vi "Write Self-Test.vi"(8 "error in (no error)":errorcluster, 10 "Self-Test":bool, 11 "Selftest Device Msg in":refnum<class "Selftest Device Msg.lvclass">) -> (0 "error out":errorcluster, 3 "Selftest Device Msg out":refnum<class "Selftest Device Msg.lvclass">)   [LabVIEW 2016, in "CS++DeviceActor.lvlib" / "Selftest Device Msg.lvclass"]
uses:
  Selftest Device Msg.lvclass
  Selftest Device Msg.lvclass/Selftest Device Msg.ctl
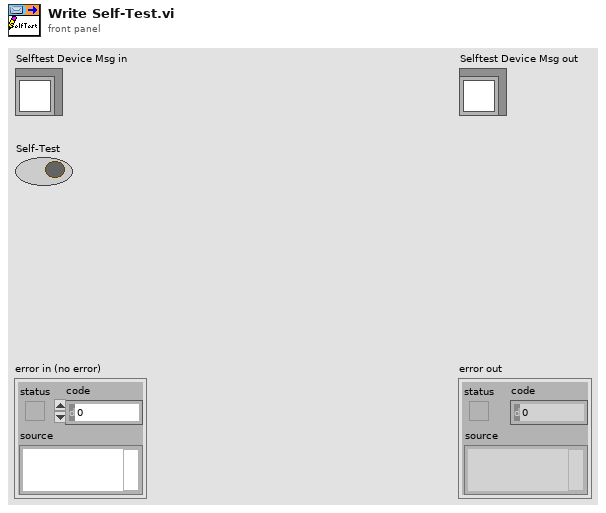
[diagram p1: front panel]
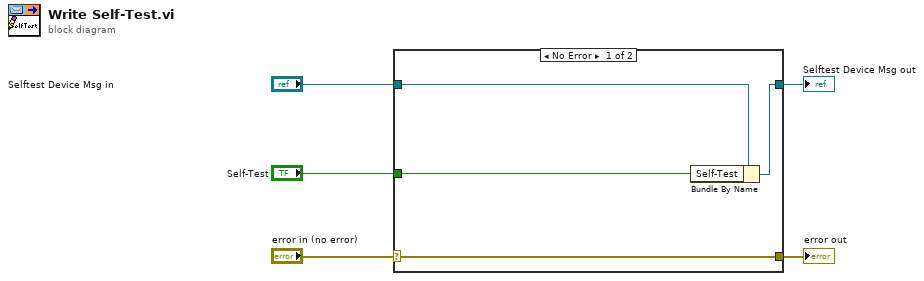
[diagram p0: block diagram]
diagram:
  n1 = case shown="No Error" "error in (no error)" {
    selector: "error in (no error)" -> [w9 w10]
    tunnel: [w9 w10] -> w4
    tunnel: [w7 w11] -> w2
    tunnel: "Selftest Device Msg in" -> [w8 w11]
    tunnel: "Self-Test" -> [w6 _]
    frame No Error {
      n2 = Bundle By Name(cluster=w8, "Self-Test"=w6) -> (w7:refnum<class "Selftest Device Msg.lvclass">)
    }
    frame Error {
    }
  }
  "error out" <- w4
  "Selftest Device Msg out" <- w2
